vi "MeasuringDevice.Measure.vi"(8 "error in (no error)":errorcluster, 11 "SMU in":refnum<class "SMU.lvclass">) -> (0 "error out":errorcluster, 2 "Result":variant, 3 "SMU out":refnum<class "SMU.lvclass">)   [LabVIEW 2017, in "SMU.lvclass"]
doc: "---------------------------------------------------------------\nJKI State Machine Objects™\nhttp://jki.net/state-machine-objects/\nCopyright (C) 2005-2015, JKI <info@jki.net>\nALL RIGHTS RESERVEDJKI State Machine Objects (SMO) 1.0.0.5\nJKI - JKI\nCopyright (c) 2016, JKI"
uses:
  SMU.lvclass
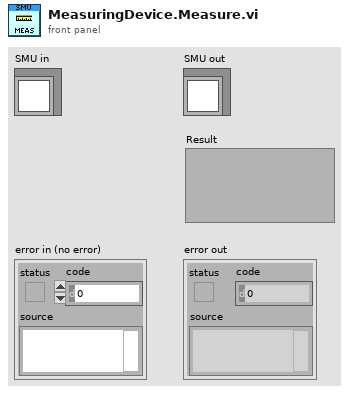
[diagram p1: front panel]
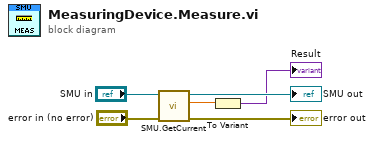
[diagram p0: block diagram]
diagram:
  n1 = call-dynamic "SMU.GetCurrent.vi"("error in (no error)"="error in (no error)", "SMU in"="SMU in") -> ("error out"=→"error out":errorcluster, "Current, A"=w4:dbl, "SMU out"=→"SMU out":refnum<class "SMU.lvclass">)  [unwired: 7 in]
  n2 = To Variant(anything=w4) -> (Variant=→"Result":variant)
